vi "example_02_xml_to_json.vi"() -> ()   [LabVIEW 2015, in "lv-unit-conversion.lvlib"]
uses:
  lv-unit-conversion.lvlib
  public/advanced/load_dictionary_xml.vi
  public/advanced/save_dictionary_json.vi
panel:
  in  "symbols []":string[](array[string])
  out "unit_dictionary":variant
  out "error out":errorcluster
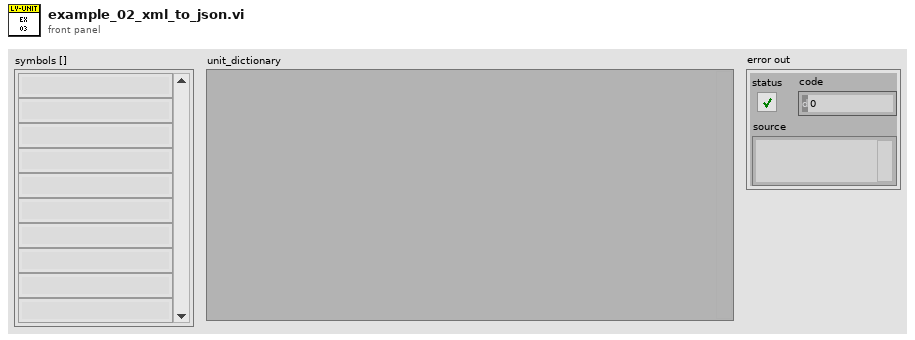
[diagram p1: front panel]
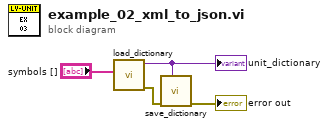
[diagram p0: block diagram]
diagram:
  n1 = call-poly "load_dictionary.vi"("symbols []"="symbols []") -> ("error out"=w3:errorcluster, "unit_dictionary"=w2:variant)  [unwired: 9 in]
  "unit_dictionary" <- w2
  n2 = call-poly "save_dictionary.vi"("unit_dictionary"=w2, "error in (no error)"=w3) -> ("error out"=→"error out":errorcluster)  [unwired: 9 in]
